vi "TwoPinsTwoInstrumentTypesOneSiteReservation_CallGetConnectionFromPin_ReturnsOneConnection.vi"(8 "error in":errorcluster) -> (0 "error out":errorcluster, 2 "result":string, 3 "pass":bool)   [LabVIEW 2020, in "MeasurementServerTests.lvlib"]
uses:
  MeasurementServerTests.lvlib
  Runtime/MeasurementLink Session Management/Session Reservation/Connection.ctl
  Runtime/MeasurementLink Session Management/Session Reservation/Hardware Independent Connection.ctl
  c3cb69a0-23cd-49fc-99d1-8c54773f0200.vi
  b3e5c3be-b7a7-4b6e-86ee-709eea9cb752.vi
  Runtime/MeasurementLink Session Management/Session Reservation/Get Connections Impl.vi
  Runtime/MeasurementLink Session Management/Session Reservation/Session Reservation.lvclass
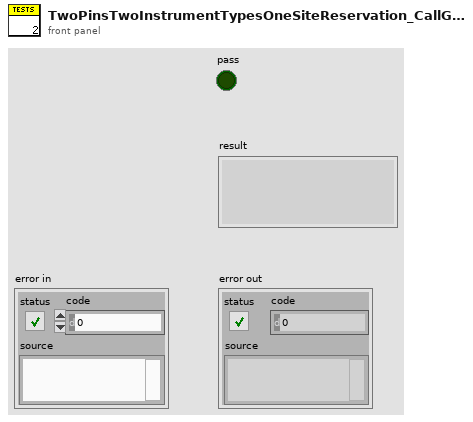
[diagram p1: front panel]
types:
  T1 = typedef "MeasurementLink Session Management.lvlib/Session Reservation.lvclass/Connection.ctl" = cluster{"connection":T2, "session":variant}
  T2 = typedef "MeasurementLink Session Management.lvlib/Session Reservation.lvclass/Hardware Independent Connection.ctl" = cluster{"pin or relay name":string, "site":i32, "instrument type id":string, "channel":string}
  T3 = typedef "MeasurementLink Session Management Client.lvlib/ni_measurementlink_sessionmanagement_v1_ChannelMapping.ctl" = cluster{"pin_or_relay_name":string, "site":i32, "channel":string}
  T4 = typedef "MeasurementLink Session Management.lvlib/Session Reservation.lvclass/Data.ctl" = cluster{"session and driver infos":T5[], "pins":string[]}
  T5 = typedef "MeasurementLink Session Management.lvlib/Session Reservation.lvclass/Session and Driver Info.ctl" = cluster{"session info":T6, "session created":bool, "session":variant}
  T6 = typedef "MeasurementLink Session Management Client.lvlib/ni_measurementlink_sessionmanagement_v1_SessionInformation.ctl" = cluster{"session":T7, "resource_name":string, "channel_list":string, "instrument_type_id":string, "session_exists":bool, "channel_mappings":T3[]}
  T7 = typedef "MeasurementLink Session Management Client.lvlib/nidevice_grpc_Session.ctl" = cluster{"name":string}
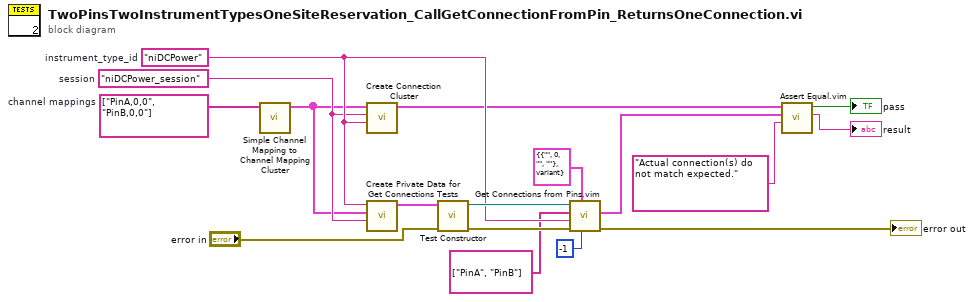
[diagram p0: block diagram]
diagram:
  w5 = string[] ["PinA,0,0", "PinB,0,0"]  # channel mappings
  w9 = "niDCPower_session"  # session
  w10 = "niDCPower"  # instrument_type_id
  n1 = call "Simple Channel Mapping to Channel Mapping Cluster.vi"("simple channel mappings"=w5) -> ("channel mappings"=w4:T3[])  [unwired: 10 in]
  n2 = call "Create Connection Cluster.vi"("instrument_type_id"=w10, "session"=w9, "channel mappings"=w4) -> ("connections"=w2:T1[])  [unwired: 8 in]
  n3 = call "Create Private Data for Get Connections Tests.vi"("session"=w9, "channel mappings"=w4, "instrument_type_id"=w10) -> ("data"=w11:T4)  [unwired: 8 in]
  n4 = call "Test Constructor.vi"("error in"="error in", "data"=w11) -> ("error out"=w16:errorcluster, "Session Reservation out"=w15:refnum<class "Session Reservation.lvclass">)  [unwired: 8 in]
  n5 = call "Get Connections from Pins.vim"("site"=-1, "connection type"=T1 {"connection"={"pin or relay name"="", "site"=0, "instrument type id"="", "channel"=""}, "session"=variant} ("connection"), "error in"=w16, "instrument type id"=w10, "pin or relay names"=string[] ["PinA", "PinB"], "session reservation in"=w15) -> ("error out"=→"error out":errorcluster, "connections"=w8:T1[])  [unwired: 3 in, 1 out]
  n6 = call "Assert Equal.vim"("failure message"="Actual connection(s) do not match expected.", "actual value"=w8, "expected value"=w2) -> ("message"=→"result":string, "equal?"=→"pass":bool)  [unwired: 7 in]
